vi "Slack-Exchange Code For Identity Token.vi"(0 "code":string, 5 "client_id":string="1023330033985.1023512746241", 7 "client_secret":string="62f876b60829c507c6cb25bfe9dbba2b", 11 "error in (no error)":errorcluster) -> (4 "access_token":string, 15 "error out":errorcluster)   [LabVIEW 2020]
uses:
  <vilib>/httpClient/POSTBuffer.vi
  <vilib>/httpClient/LabVIEWHTTPClient.lvlib
panel:
  out "body":string
  out "headers":string
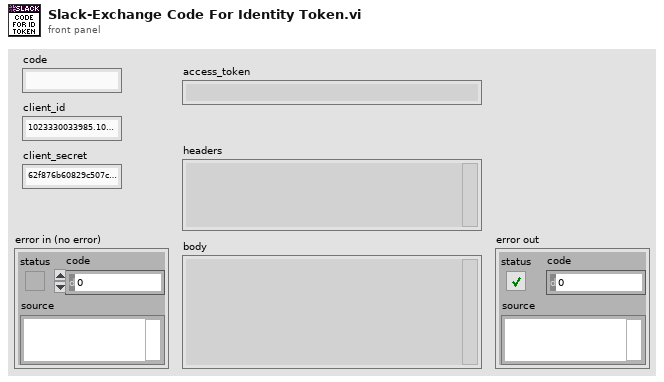
[diagram p1: front panel]
types:
  T1 = cluster{"ok":bool, "access_token":string, "scope":string, "team_id":string}
  T2 = typedef "LabVIEWHTTPClient.lvlib/ClientHandle.ctl" = refnum<k1>
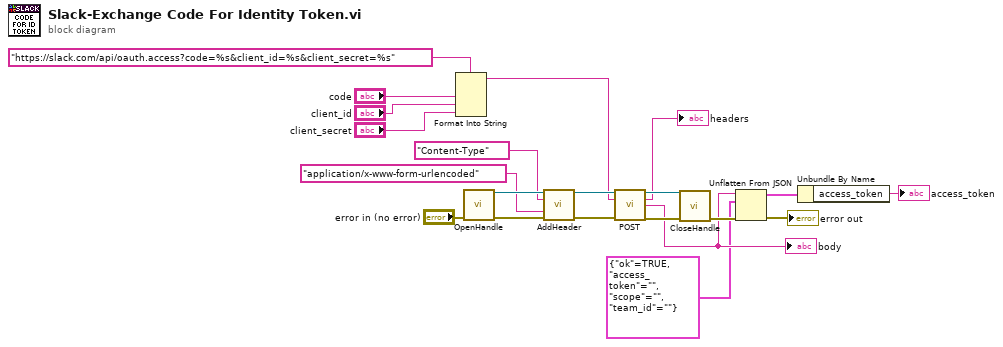
[diagram p0: block diagram]
diagram:
  n1 = Format Into String(format string="https://slack.com/api/oauth.access?code=%s&client_id=%s&client_secret=%s", "code", "client_id", "client_secret") -> (resulting string=w13:string)  [unwired: 2 in, 1 out]
  n2 = call <vilib>:"OpenHandle.vi"("error in (no error)"="error in (no error)") -> ("client handle out"=w20:T2, "error out"=w21:errorcluster)  [unwired: 13 in]
  n3 = call <vilib>:"AddHeader.vi"("client handle"=w20, "header"="Content-Type", "value"="application/x-www-form-urlencoded", "error in (no error)"=w21) -> ("client handle out"=w16:T2, "error out"=w17:errorcluster)  [unwired: 10 in]
  n4 = call-poly <vilib>:"POST.vi"("client handle"=w16, "url"=w13, "error in (no error)"=w17) -> ("client handle out"=w12:T2, "headers"=→"headers":string, "body"=w4:string, "error out"=w11:errorcluster)  [unwired: 9 in]
  "body" <- w4
  n5 = call <vilib>:"CloseHandle.vi"("client handle"=w12, "error in (no error)"=w11) -> ("error out"=w6:errorcluster)  [unwired: 13 in]
  n6 = Unflatten From JSON(JSON string=w4, type and defaults=T1 {"ok"=TRUE, "access_token"="", "scope"="", "team_id"=""}, error in (no error)=w6) -> (value=w2:T1, error out=→"error out":errorcluster)  [unwired: 4 in]
  n7 = Unbundle By Name(w2) -> ("access_token"=→"access_token":string)
